vi "MainBaxterDemo.vi"() -> ()   [LabVIEW 2013]
uses:
  ROS/Code/JointPositions.ctl
  ROS/Code/SubVIs/BaxterSide.ctl
  ROS/Code/SubVIs/BaxterButtons.ctl
  ROS/Code/_ROSDefinition.vi
  BaxterVIs/Command_Joint_Angles_cluster.vi
  BaxterVIs/Read_Joint_States_A.vi
panel:
  out "ITB":T1
  in  "ITB":bool
  in  "Left Command":bool
  in  "Right":T2 {"w2" scale=-175.25..175.25; "w1" scale=-90.0..120.0; "w0" scale=-175.25..175.25; "e1" scale=-3.0..150.0; "e0" scale=-173.5..173.5; "s1" scale=-123.0..60.0; "s0" scale=-141.0..51.0}
  out "Active Servers":T3(array[cluster])
  in  "kill":bool
  out "Port Count":i32
  in  "Gripper":T4(radio)=enum."Calibrate"
  out "Left":u32
  out "Right":u32
  in  "Load Joints":bool
  in  "Pan":bool
  in  "target":sgl(slide) scale=-1.0..1.0
  out "Initialized":bool
  in  "IR Sensors":bool
  in  "Right Command":bool
  in  "Joint Status":bool
  in  "Nod":bool
  in  "Left":T2 {"w2" scale=-175.25..175.25; "w1" scale=-90.0..120.0; "w0" scale=-175.25..175.25; "e1" scale=-3.0..150.0; "e0" scale=-173.5..173.5; "s1" scale=-123.0..60.0; "s0" scale=-141.0..51.0}
  out "Joint States":T5(array[cluster])
  in  "disconnect head topic":bool
  in  "stop":bool
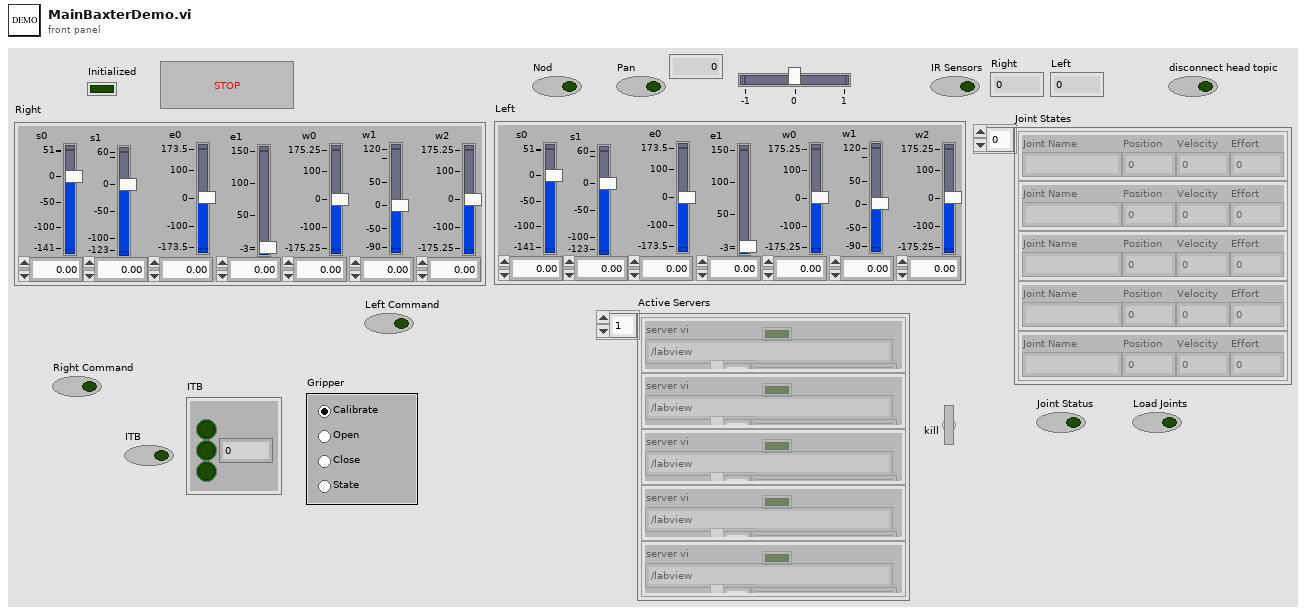
[diagram p1: front panel]
types:
  T1 = cluster{"Top":bool, "Wheel":bool, "Bottom":bool, "Wheel":u8}
  T2 = typedef "JointPositions.ctl" = cluster{"e0":dbl, "e1":dbl, "s0":dbl, "s1":dbl, "w0":dbl, "w1":dbl, "w2":dbl}
  T3 = cluster{"server vi":string, "reference":refnum<vi>, "Description":string[], "Connected":bool}[]
  T4 = enum32{"No Selection", "Calibrate", "Open", "Close", "State"}
  T5 = cluster{"Joint Name":string, "Position":dbl, "Velocity":dbl, "Effort":dbl}[]
  T6 = typedef "BaxterSide.ctl" = enum16{"left", "right"}
  T7 = typedef "BaxterButtons.ctl" = u16
  T8 = cluster{"Cancel":bool, "OK":bool, "Show":bool, "Wheel":u8}
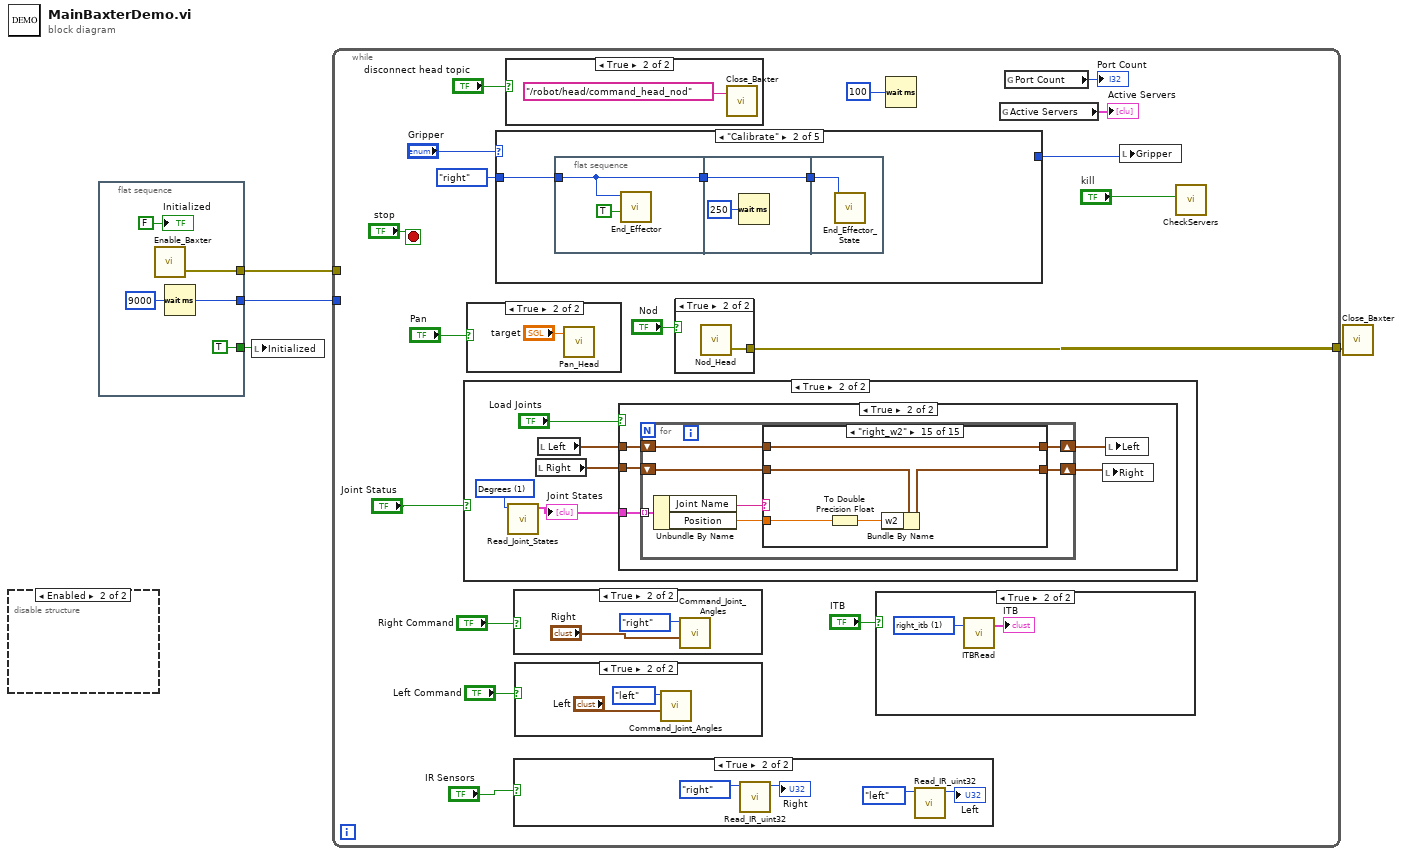
[diagram p0: block diagram]
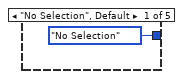
[diagram p5: hidden frame]
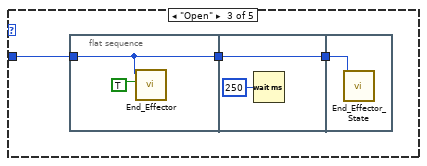
[diagram p6: hidden frame]
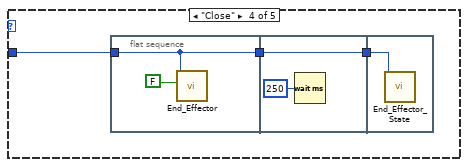
[diagram p7: hidden frame]
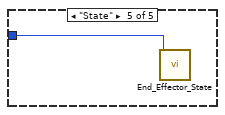
[diagram p8: hidden frame]
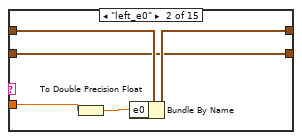
[diagram p14: hidden frame]
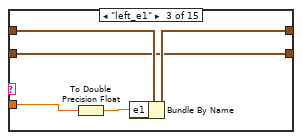
[diagram p15: hidden frame]
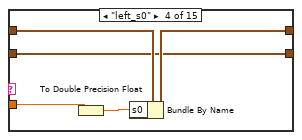
[diagram p16: hidden frame]
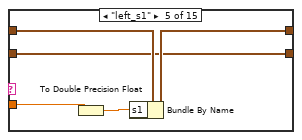
[diagram p17: hidden frame]
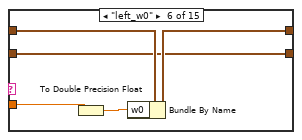
[diagram p18: hidden frame]
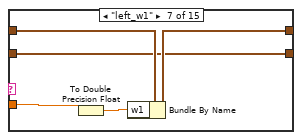
[diagram p19: hidden frame]
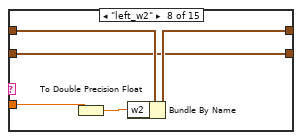
[diagram p20: hidden frame]
diagram:
  n1 = disable-structure shown="Enabled" {
    frame Disabled {
      n2 = global read "_ROSDefinition.vi" "Nodes"() -> ()  [unwired: 1 out]
      n3 = call "_ROSMasterConsole.vi"() -> ()  [unwired: 12 in]
    }
    frame Enabled {
    }
  }
  n4 = flat-sequence {
    tunnel: [w9] -> w3
    tunnel: [w7] -> w2
    tunnel: [TRUE] -> w1
    frame #0 {
      n5 = call "Enable_Baxter.vi"() -> ("error out"=w9:errorcluster)  [unwired: 4 in]
      n6 = Wait (ms)(milliseconds to wait=u32 9000) -> (millisecond timer value=w7:u32)
      "Initialized" <- FALSE ("Initialized")
    }
  }
  n7 = local write "Initialized"(w1) -> ()
  n8 = while {
    tunnel: [w19] -> w4
    tunnel: w3 -> [_]
    tunnel: w2 -> [_]
    stop <- "stop" stop-if-true
    n9 = case shown="True" "Joint Status" {
      frame False {
      }
      frame True {
        w68 = u16 1 items=["Radians", "Degrees"] ("Units (Rad)")
        n10 = call-poly "Read_Joint_States.vi"("Units (deg)"=w68) -> ("Joint States"=w66:T5)  [unwired: 4 in, 3 out]
        "Joint States" <- w66
        n11 = local read "Right"() -> (w64:T2)
        n12 = local read "Left"() -> (w65:T2)
        n13 = case shown="True" "Load Joints" {
          tunnel: w66 -> [_ w73]
          tunnel: w65 -> [_ w72]
          tunnel: w64 -> [_ w70]
          frame False {
          }
          frame True {
            n14 = for {
              tunnel: w73 -> [w80] mode=indexing
              shift-right: [w79] -> w71
              shift-left: w72 -> [w78]
              shift-right: [w74] -> w69
              shift-left: w70 -> [w75]
              n15 = Unbundle By Name(w80) -> ("Joint Name"=w77:string, "Position"=w76:dbl)
              n16 = case shown="\"right_w2\"" w77 {
                tunnel: [w82 w87 w92 w97 w102 w107 w112 w117 w118 w123 w128 w133 w138 w143 w148] -> w79
                tunnel: w78 -> [w82 w86 w91 w96 w101 w106 w111 w116 w118 w123 w128 w133 w138 w143 w148]
                tunnel: w76 -> [_ w84 w89 w94 w99 w104 w109 w114 w121 w126 w131 w136 w141 w146 w151]
                tunnel: w75 -> [w81 w83 w88 w93 w98 w103 w108 w113 w120 w125 w130 w135 w140 w145 w150]
                tunnel: [w81 w83 w88 w93 w98 w103 w108 w113 w119 w124 w129 w134 w139 w144 w149] -> w74
                frame Default {
                }
                frame "left_e0" {
                  n17 = To Double Precision Float(number=w84) -> (double precision float=w85:dbl)
                  n18 = Bundle By Name(cluster=w86, "e0"=w85) -> (w87:T2)
                }
                frame "left_e1" {
                  n19 = To Double Precision Float(number=w89) -> (double precision float=w90:dbl)
                  n20 = Bundle By Name(cluster=w91, "e1"=w90) -> (w92:T2)
                }
                frame "left_s0" {
                  n21 = To Double Precision Float(number=w94) -> (double precision float=w95:dbl)
                  n22 = Bundle By Name(cluster=w96, "s0"=w95) -> (w97:T2)
                }
                frame "left_s1" {
                  n23 = To Double Precision Float(number=w99) -> (double precision float=w100:dbl)
                  n24 = Bundle By Name(cluster=w101, "s1"=w100) -> (w102:T2)
                }
                frame "left_w0" {
                  n25 = To Double Precision Float(number=w104) -> (double precision float=w105:dbl)
                  n26 = Bundle By Name(cluster=w106, "w0"=w105) -> (w107:T2)
                }
                frame "left_w1" {
                  n27 = To Double Precision Float(number=w109) -> (double precision float=w110:dbl)
                  n28 = Bundle By Name(cluster=w111, "w1"=w110) -> (w112:T2)
                }
                frame "left_w2" {
                  n29 = To Double Precision Float(number=w114) -> (double precision float=w115:dbl)
                  n30 = Bundle By Name(cluster=w116, "w2"=w115) -> (w117:T2)
                }
                frame "right_e0" {
                  n31 = To Double Precision Float(number=w121) -> (double precision float=w122:dbl)
                  n32 = Bundle By Name(cluster=w120, "e0"=w122) -> (w119:T2)
                }
                frame "right_e1" {
                  n33 = To Double Precision Float(number=w126) -> (double precision float=w127:dbl)
                  n34 = Bundle By Name(cluster=w125, "e1"=w127) -> (w124:T2)
                }
                frame "right_s0" {
                  n35 = To Double Precision Float(number=w131) -> (double precision float=w132:dbl)
                  n36 = Bundle By Name(cluster=w130, "s0"=w132) -> (w129:T2)
                }
                frame "right_s1" {
                  n37 = To Double Precision Float(number=w136) -> (double precision float=w137:dbl)
                  n38 = Bundle By Name(cluster=w135, "s1"=w137) -> (w134:T2)
                }
                frame "right_w0" {
                  n39 = To Double Precision Float(number=w141) -> (double precision float=w142:dbl)
                  n40 = Bundle By Name(cluster=w140, "w0"=w142) -> (w139:T2)
                }
                frame "right_w1" {
                  n41 = To Double Precision Float(number=w146) -> (double precision float=w147:dbl)
                  n42 = Bundle By Name(cluster=w145, "w1"=w147) -> (w144:T2)
                }
                frame "right_w2" {
                  n43 = To Double Precision Float(number=w151) -> (double precision float=w152:dbl)
                  n44 = Bundle By Name(cluster=w150, "w2"=w152) -> (w149:T2)
                }
              }
            }
            n45 = local write "Right"(w69) -> ()
            n46 = local write "Left"(w71) -> ()
          }
        }
      }
    }
    n47 = case shown="True" "Pan" {
      frame False {
      }
      frame True {
        n48 = call "Pan_Head.vi"("target"="target") -> ()  [unwired: 4 in, 1 out]
      }
    }
    n49 = case shown="\"Calibrate\"" "Gripper" {
      tunnel: [T4."No Selection" ("Gripper") _ _ _ _] -> w16
      tunnel: BaxterSide."right" ("Side") -> [_ w35 w43 w51 w57]
      frame "No Selection", Default {
      }
      frame "Calibrate" {
        n50 = flat-sequence {
          tunnel: w35 -> [w36]
          tunnel: [w36] -> w33
          tunnel: [w38] -> w34
          tunnel: w33 -> [w38]
          tunnel: w34 -> [w40]
          frame #0 {
            n51 = call "End_Effector.vi"("Calibrate"=TRUE, "Side"=w36) -> ()  [unwired: 6 in, 1 out]
          }
          frame #1 {
            n52 = Wait (ms)(milliseconds to wait=u32 250) -> ()  [unwired: 1 out]
          }
          frame #2 {
            n53 = call "End_Effector_State.vi"("Side"=w40) -> ()  [unwired: 6 in, 2 out]
          }
        }
      }
      frame "Open" {
        n54 = flat-sequence {
          tunnel: w43 -> [w44]
          tunnel: [w44] -> w42
          tunnel: w42 -> [w46]
          tunnel: [w46] -> w41
          tunnel: w41 -> [w48]
          frame #0 {
            n55 = call "End_Effector.vi"("Open"=TRUE ("Calibrate"), "Side"=w44) -> ()  [unwired: 6 in, 1 out]
          }
          frame #1 {
            n56 = Wait (ms)(milliseconds to wait=u32 250) -> ()  [unwired: 1 out]
          }
          frame #2 {
            n57 = call "End_Effector_State.vi"("Side"=w48) -> ()  [unwired: 6 in, 2 out]
          }
        }
      }
      frame "Close" {
        n58 = flat-sequence {
          tunnel: w51 -> [w52]
          tunnel: [w52] -> w49
          tunnel: [w54] -> w50
          tunnel: w49 -> [w54]
          tunnel: w50 -> [w56]
          frame #0 {
            n59 = call "End_Effector.vi"("Open"=FALSE ("Calibrate"), "Side"=w52) -> ()  [unwired: 6 in, 1 out]
          }
          frame #1 {
            n60 = Wait (ms)(milliseconds to wait=u32 250) -> ()  [unwired: 1 out]
          }
          frame #2 {
            n61 = call "End_Effector_State.vi"("Side"=w56) -> ()  [unwired: 6 in, 2 out]
          }
        }
      }
      frame "State" {
        n62 = call "End_Effector_State.vi"("Side"=w57) -> ()  [unwired: 6 in, 2 out]
      }
    }
    n63 = case shown="True" "disconnect head topic" {
      frame False {
      }
      frame True {
        n64 = call "Close_Baxter.vi"("topic"="/robot/head/command_head_nod") -> ()  [unwired: 3 in, 1 out]
      }
    }
    n65 = case shown="True" "Right Command" {
      frame False {
      }
      frame True {
        n66 = call-poly "Command_Joint_Angles.vi"("Arm Angles (degrees)"="Right", "Side"=BaxterSide."right") -> ()  [unwired: 7 in, 1 out]
      }
    }
    n67 = case shown="True" "IR Sensors" {
      frame False {
      }
      frame True {
        n68 = call "Read_IR_uint32.vi"("Side"=BaxterSide."right") -> ("Range"=→"Right":u32)  [unwired: 4 in, 3 out]
        n69 = call "Read_IR_uint32.vi"("Side"=BaxterSide."left") -> ("Range"=→"Left":u32)  [unwired: 4 in, 3 out]
      }
    }
    n70 = case shown="True" "Left Command" {
      frame False {
      }
      frame True {
        n71 = call-poly "Command_Joint_Angles.vi"("Arm Angles (degrees)"="Left", "Side"=BaxterSide."left") -> ()  [unwired: 7 in, 1 out]
      }
    }
    n72 = case shown="True" "Nod" {
      tunnel: [_ w154] -> w19
      frame False {
      }
      frame True {
        n73 = call "Nod_Head.vi"() -> ("error out"=w154:errorcluster)  [unwired: 4 in]
      }
    }
    n74 = case shown="True" "ITB" {
      frame False {
      }
      frame True {
        w28 = T7 1 items=["left_itb", "right_itb", "torso_left_itb", "torso_right_itb"] ("Component")
        n75 = call "ITBRead.vi"("Component"=w28) -> ("ITB"=→"ITB":T8)  [unwired: 2 in, 1 out]
      }
    }
    n76 = Wait (ms)(milliseconds to wait=u32 100) -> ()  [unwired: 1 out]
    n77 = global read "_ROSDefinition.vi" "Active Servers"() -> (→"Active Servers":T3)
    n78 = global read "_ROSDefinition.vi" "Port Count"() -> (→"Port Count":i32)
    n79 = local write "Gripper"(w16) -> ()
    n80 = call "CheckServers.vi"("kill"="kill") -> ()  [unwired: 11 in]
  }
  n81 = call "Close_Baxter.vi"("error in"=w4) -> ()  [unwired: 3 in, 1 out]
